vi "Score Goal.vi"(8 "error in (no error)":errorcluster, 9 "Speed":dbl, 10 "Team Blue?":bool) -> (0 "error out":errorcluster)   [LabVIEW 2016]
uses:
  <vilib>/Rock Robotics/WPI/RobotDrive/WPI_RobotDriveMecanumDrive_Cartesian.vi
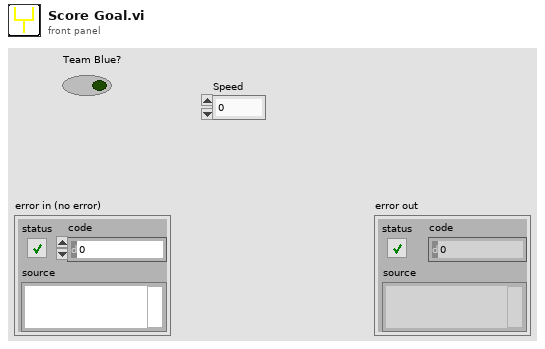
[diagram p1: front panel]
types:
  T1 = typedef "WPI_RobotDriveDevRef.ctl" = cluster{"DevStatus":errorcluster, "Motors[]":T2[], "Square Inputs":bool, "Max Output":dbl}
  T2 = typedef "WPI_MotorControlDeviceRef.ctl" = cluster{"DeviceStatus":errorcluster, "Type":T3, "PWM":cluster{"PWM Channel":T4, "DeadBand":T5}, "CAN":cluster{"Device Number":u8, "SetOutput VI Ref":variant, "GetOutput VI Ref":variant, "Enable VI Ref":variant, "Disable VI Ref":variant, "Data":variant}, "Invert":bool}
  T3 = typedef "WPI_MotorControlType.ctl" = enum16{"PWM", "CAN"}
  T4 = typedef "FPGA_DIOPWMChannel.ctl" = enum8{"PWM 0", "PWM 1", "PWM 2", "PWM 3", "PWM 4", "PWM 5", "PWM 6", "PWM 7", "PWM 8", "PWM 9", "PWM MXP 0", "PWM MXP 1", "PWM MXP 2", "PWM MXP 3", "PWM MXP 4", "PWM MXP 5", "PWM MXP 6", "PWM MXP 7", "PWM MXP 8", "PWM MXP 9", "Invalid"}
  T5 = typedef "WPI_PWMDeadband.ctl" = cluster{"Name":string, "maxPositivePwm":i32, "minPositivePwm":i32, "centerPwm":i32, "maxNegativePwm":i32, "minNegativePwm":i32, "angularRange":u16}
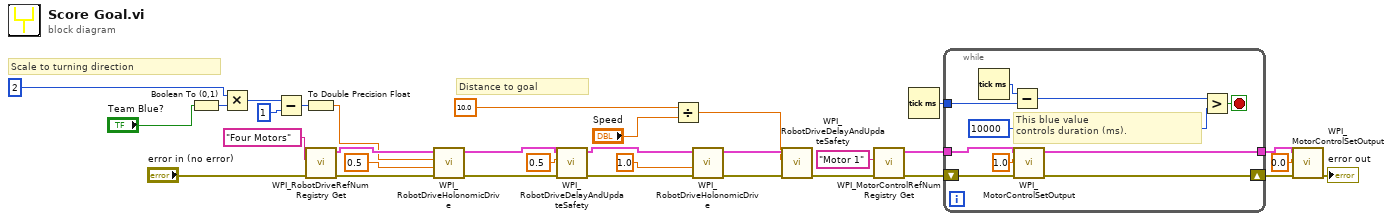
[diagram p0: block diagram]
diagram:
  # "Distance to goal"
  # "Scale to turning direction"
  n1 = Boolean To (0,1)(Boolean="Team Blue?") -> (0, 1=w22:i16)
  n2 = Multiply(x=i16 2, y=w22) -> (x*y=w20:i16)
  n3 = Subtract(x=w20, y=i16 1) -> (x-y=w19:i16)
  n4 = To Double Precision Float(number=w19) -> (double precision float=w18:dbl)
  n5 = call <vilib>:"WPI_RobotDriveRefNum Registry Get.vi"("error in (no error)"="error in (no error)", "refnum name"="Four Motors") -> ("error out"=w30:errorcluster, "RobotDriveDevRef"=w29:T1)  [unwired: 8 in]
  n6 = call-poly <vilib>:"WPI_RobotDriveHolonomicDrive.vi"("error in (no error)"=w30, "Y"=0.5, "X"=w18, "RobotDriveDevRef"=w29) -> ("error out"=w26:errorcluster, "RobotDriveDevRef"=w27:T1)  [unwired: 5 in, 1 out]
  n7 = call <vilib>:"WPI_RobotDriveDelayAndUpdateSafety.vi"("error in (no error)"=w26, "Delay (s)"=0.5, "RobotDriveDevRef"=w27) -> ("error out"=w17:errorcluster, "RobotDriveDevRef 2"=w16:T1)  [unwired: 7 in]
  n8 = Divide(x=10.0, y="Speed") -> (x/y=w10:dbl)
  n9 = call-poly <vilib>:"WPI_RobotDriveHolonomicDrive.vi"("error in (no error)"=w17, "Y"=1.0, "RobotDriveDevRef"=w16) -> ("error out"=w14:errorcluster, "RobotDriveDevRef"=w13:T1)  [unwired: 6 in, 1 out]
  n10 = call <vilib>:"WPI_RobotDriveDelayAndUpdateSafety.vi"("error in (no error)"=w14, "Delay (s)"=w10, "RobotDriveDevRef"=w13) -> ("error out"=w9:errorcluster)  [unwired: 7 in, 1 out]
  n11 = call <vilib>:"WPI_MotorControlRefNum Registry Get.vi"("error in (no error)"=w9, "refnum name"="Motor 1") -> ("error out"=w7:errorcluster, "MotorControlDevRef"=w6:T2)  [unwired: 8 in]
  n12 = Tick Count (ms)() -> (millisecond timer value=w5:u32)
  n13 = while {
    tunnel: w6 -> [w41]
    shift-right: [w39] -> w4
    shift-left: w7 -> [w42]
    tunnel: w5 -> [w37]
    tunnel: [w33] -> w3
    stop <- w34 stop-if-true
    # "This blue value\ncontrols duration (ms)."
    n14 = Tick Count (ms)() -> (millisecond timer value=w38:u32)
    n15 = Subtract(x=w38, y=w37) -> (x-y=w36:u32)
    n16 = call <vilib>:"WPI_MotorControlSetOutput.vi"("error in (no error)"=w42, "Output"=1.0, "MotorControlDevRef"=w41) -> ("error out"=w39:errorcluster, "MotorControlDevRef"=w33:T2)  [unwired: 6 in, 1 out]
    n17 = Greater?(x=w36, y=u32 10000) -> (0:w34:bool)
  }
  n18 = call <vilib>:"WPI_MotorControlSetOutput.vi"("error in (no error)"=w4, "Output"=0.0, "MotorControlDevRef"=w3) -> ("error out"=→"error out":errorcluster)  [unwired: 6 in, 2 out]
